vi "getData.vi"(11 "Filled Text Fields Actor in":refnum<class "Filled Text Fields Actor.lvclass">) -> (2 "Data":string, 3 "Filled Text Fields Actor out":refnum<class "Filled Text Fields Actor.lvclass">)   [LabVIEW 2017, in "Filled Text Fields.lvlib" / "Filled Text Fields Actor.lvclass"]
uses:
  Filled Text Fields Actor.lvclass
  Filled Text Fields Actor.lvclass/Filled Text Fields Actor.ctl
  Data/Data.lvclass/Data.ctl
  Data/Data.lvclass
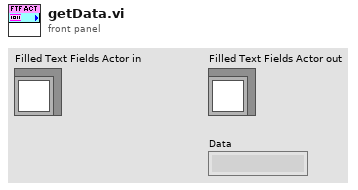
[diagram p1: front panel]
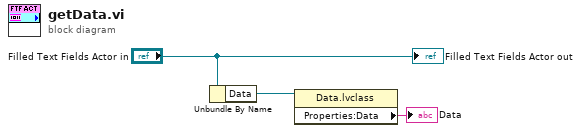
[diagram p0: block diagram]
diagram:
  n1 = Unbundle By Name("Filled Text Fields Actor in") -> ("Data"=w2:refnum<class "Data.lvclass">)
  n2 = property class="Data.lvclass"(reference=w2) -> ("Properties:Data"=→"Data":string)  [unwired: 1 in, 2 out]
  "Filled Text Fields Actor out" <- "Filled Text Fields Actor in"
